vi "Increment Iteration.vi"(8 "error in (no error)":errorcluster, 11 "Plugin in":refnum<class "Plugin.lvclass">) -> (0 "error out":errorcluster, 3 "Plugin out":refnum<class "Plugin.lvclass">)   [LabVIEW 2019, in "DSF Core.lvlib" / "Plugin.lvclass"]
uses:
  Plugin.lvclass
  Plugin.lvclass/Plugin.ctl
  Timing/Timing.lvclass
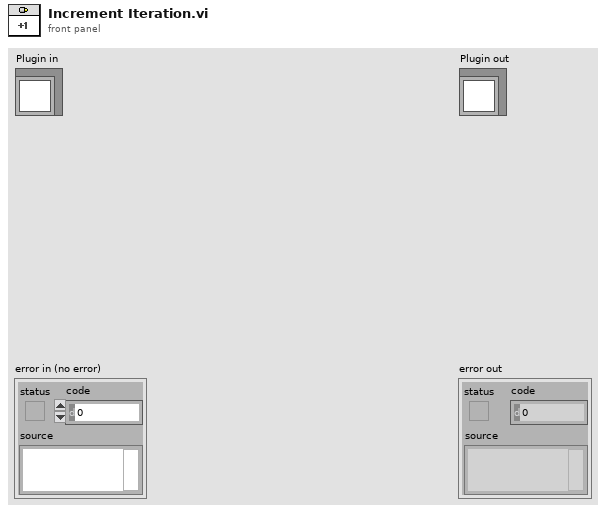
[diagram p1: front panel]
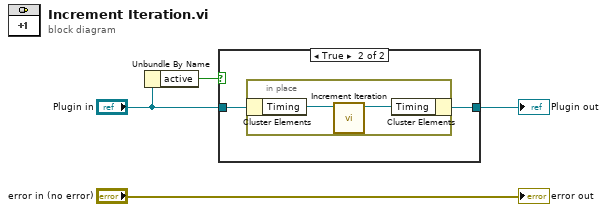
[diagram p0: block diagram]
diagram:
  n1 = Unbundle By Name("Plugin in") -> ("active"=w1:bool)
  n2 = case shown="True" w1 {
    tunnel: [w5 w7] -> w3
    tunnel: "Plugin in" -> [w5 w6]
    frame False {
    }
    frame True {
      n3 = in-place {
        n4 = in-place-cluster #1(w6) -> ("Timing"=w9:refnum<class "Timing.lvclass">)
        n5 = call "Increment Iteration.vi"("Timing in"=w9) -> ("Timing out"=w8:refnum<class "Timing.lvclass">)  [unwired: 10 in]
        n6 = in-place-cluster #1("Timing"=w8) -> (w7:refnum<class "Plugin.lvclass">)
      }
    }
  }
  "Plugin out" <- w3
  "error out" <- "error in (no error)"
